vi "MongoDB.CollectionDropIndexByName.vi"(8 "error in (no error)":errorcluster, 10 "indexName":string, 11 "MongoDB.Collection in":refnum<class "MongoDB.Collection.lvclass">) -> (0 "error out":errorcluster, 3 "MongoDB.Collection out":refnum<class "MongoDB.Collection.lvclass">)   [LabVIEW 2014, in "MongoDB.Collection.lvclass"]
uses:
  MongoDB.Collection.lvclass
  MongoDB.Collection.lvclass/MongoDB.Collection.ctl
  C:/Users/Richard/Documents/GitHub/mongo-labview-driver/CSharp/bin/MongoDB.Driver.Legacy.dll
  CSharp/bin/MongoDB.Driver.Legacy.dll
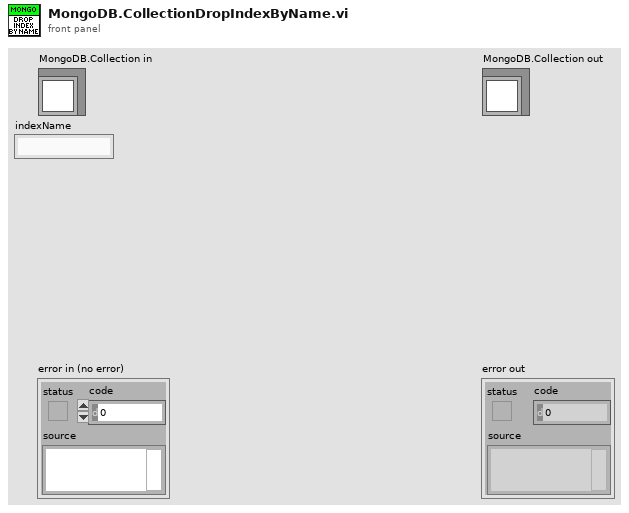
[diagram p1: front panel]
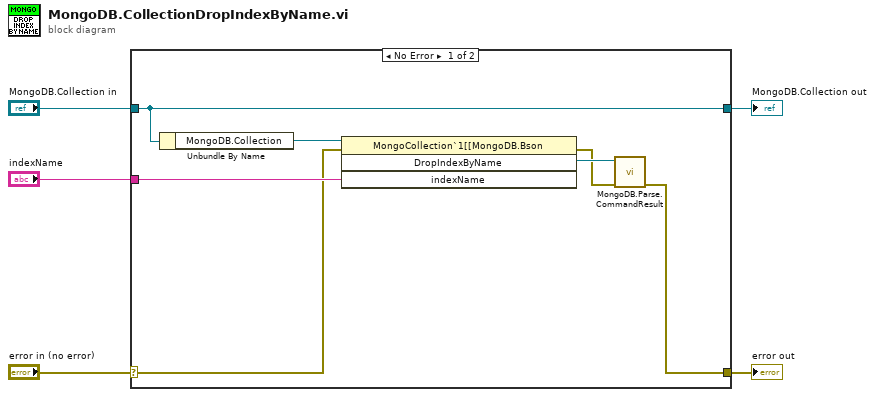
[diagram p0: block diagram]
diagram:
  n1 = case shown="No Error" "error in (no error)" {
    selector: "error in (no error)" -> [w6 w14]
    tunnel: [w7 w14] -> w4
    tunnel: [w12 w13] -> w2
    tunnel: "MongoDB.Collection in" -> [w12 w13]
    tunnel: "indexName" -> [w10 _]
    frame No Error {
      n2 = Unbundle By Name(w12) -> ("MongoDB.Collection"=w11:refnum<k24>)
      n3 = invoke class="MongoCollection`1[[MongoDB.Bson" method="DropIndexByName"(reference=w11, error in=w6, "indexName"=w10) -> (error out=w8:errorcluster, "DropIndexByName"=w9:refnum<k24>)  [unwired: 1 in, 2 out]
      n4 = call "MongoDB.Parse.CommandResult.vi"("error in (no error)"=w8, "MongoDB.Command.Result"=w9) -> ("error out"=w7:errorcluster)  [unwired: 9 in]
    }
    frame Error {
    }
  }
  "error out" <- w4
  "MongoDB.Collection out" <- w2
